vi "pulse Tx 2 spc.vi"(9 "enable line":bool=TRUE, 10 "take it!":bool, 11 "Cluster":T2={"PW"=0, "frequency shift"=0.0, "amp"=0.9999923706054688, "mode type"=enum."CW", "mode depth"=0, "mode filter"=0, "phase shift"=0.0, "pulse shape filter"=0}) -> (0 "output valid":bool, 1 "IQ out":T1[](array[typedef]), 2 "free dds":bool, 4 "frequncy":fxp<+/-,48,0>, 6 "phase":fxp<+/-,16,1>)   [LabVIEW 2021]
uses:
  pulse_tx_vis/pdw.ctl
  pulse_tx_vis/CTL/mode_type.ctl
  <instrlib>/_niInstr/DSP/v1/Shared/Public/IQ Data.ctl
  <instrlib>/_niInstr/DSP/v1/FPGA/Public/Sub VIs/Frequency Shift/Frequency Shift - 2 spc.vi
  <instrlib>/_niInstr/Basic Elements/v1/FPGA/Private/Count Up U32.vi
  <vilib>/rvi/FXPMathLib/FxpAdd/XNode/nifxpmath_Add.xnode
  <instrlib>/_niInstr/DSP/v1/Shared/niInstr DSP v1 Shared.lvlib
  <instrlib>/_niInstr/Basic Elements/v1/FPGA/niInstr Basic Elements v1 FPGA.lvlib
  <vilib>/rvi/FXPMathLib/sim/FxpSim.dll
  <instrlib>/_niInstr/DSP/v1/FPGA/niInstr DSP v1 FPGA.lvlib
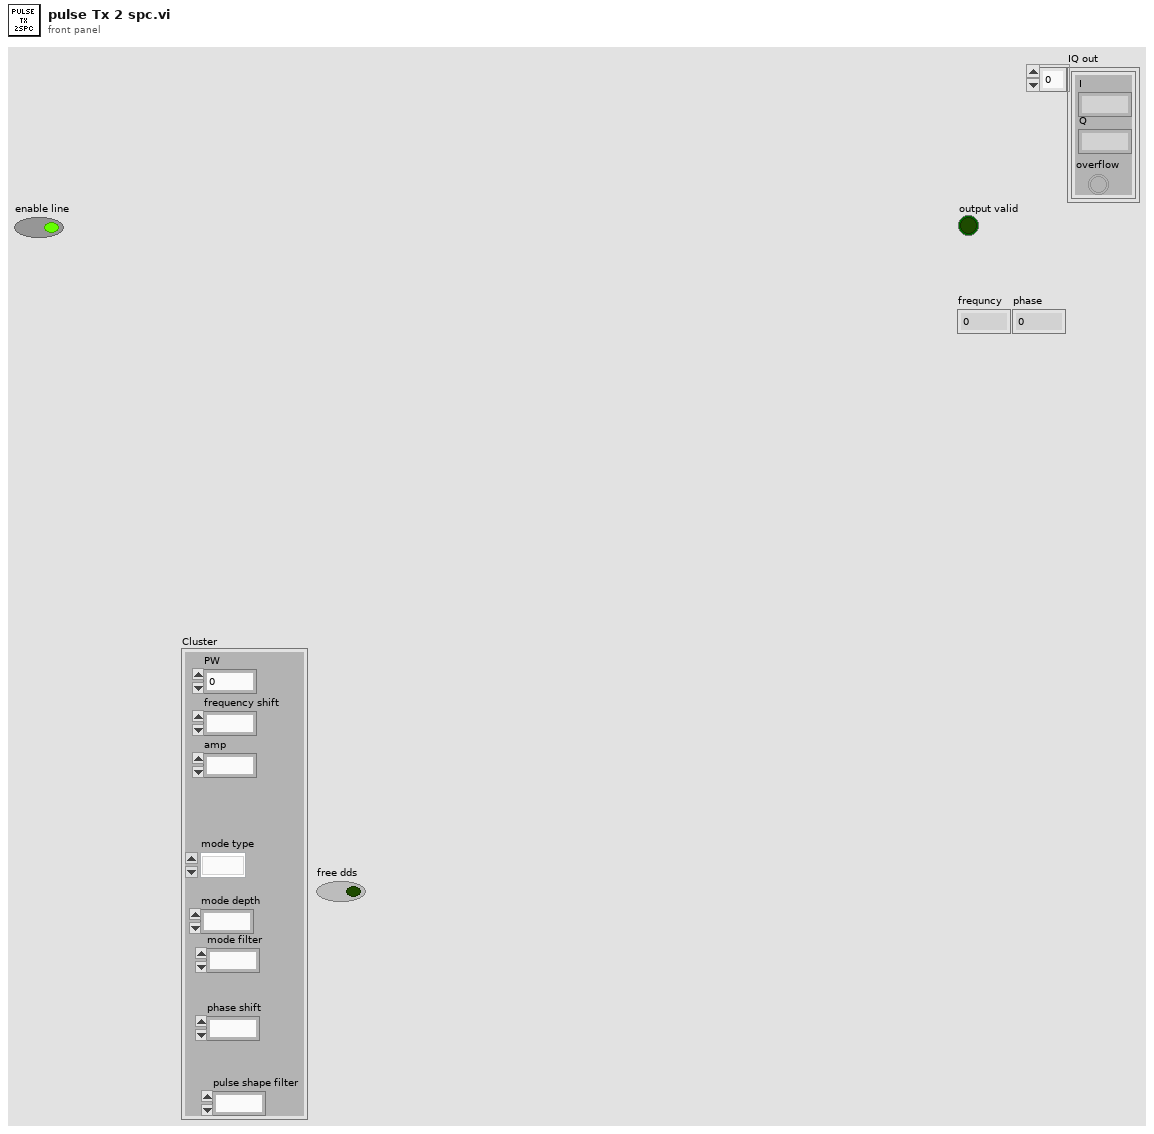
[diagram p1: front panel]
types:
  T1 = typedef "niInstr DSP v1 Shared.lvlib/IQ Data.ctl" = cluster{"I":fxp<+/-,18,1>, "Q":fxp<+/-,18,1>, "overflow":bool}
  T2 = typedef "pdw.ctl" = cluster{"PW":u32, "frequency shift":fxp<+/-,48,0>, "amp":fxp<+/-,18,1>, "mode type":T3, "mode depth":u32, "mode filter":u8, "phase shift":fxp<+/-,16,1>, "pulse shape filter":u8}
  T3 = typedef "mode_type.ctl" = enum8{"CW", "from memory 1", "NC - cw", "LFM", "BPSK", "QPSK"}
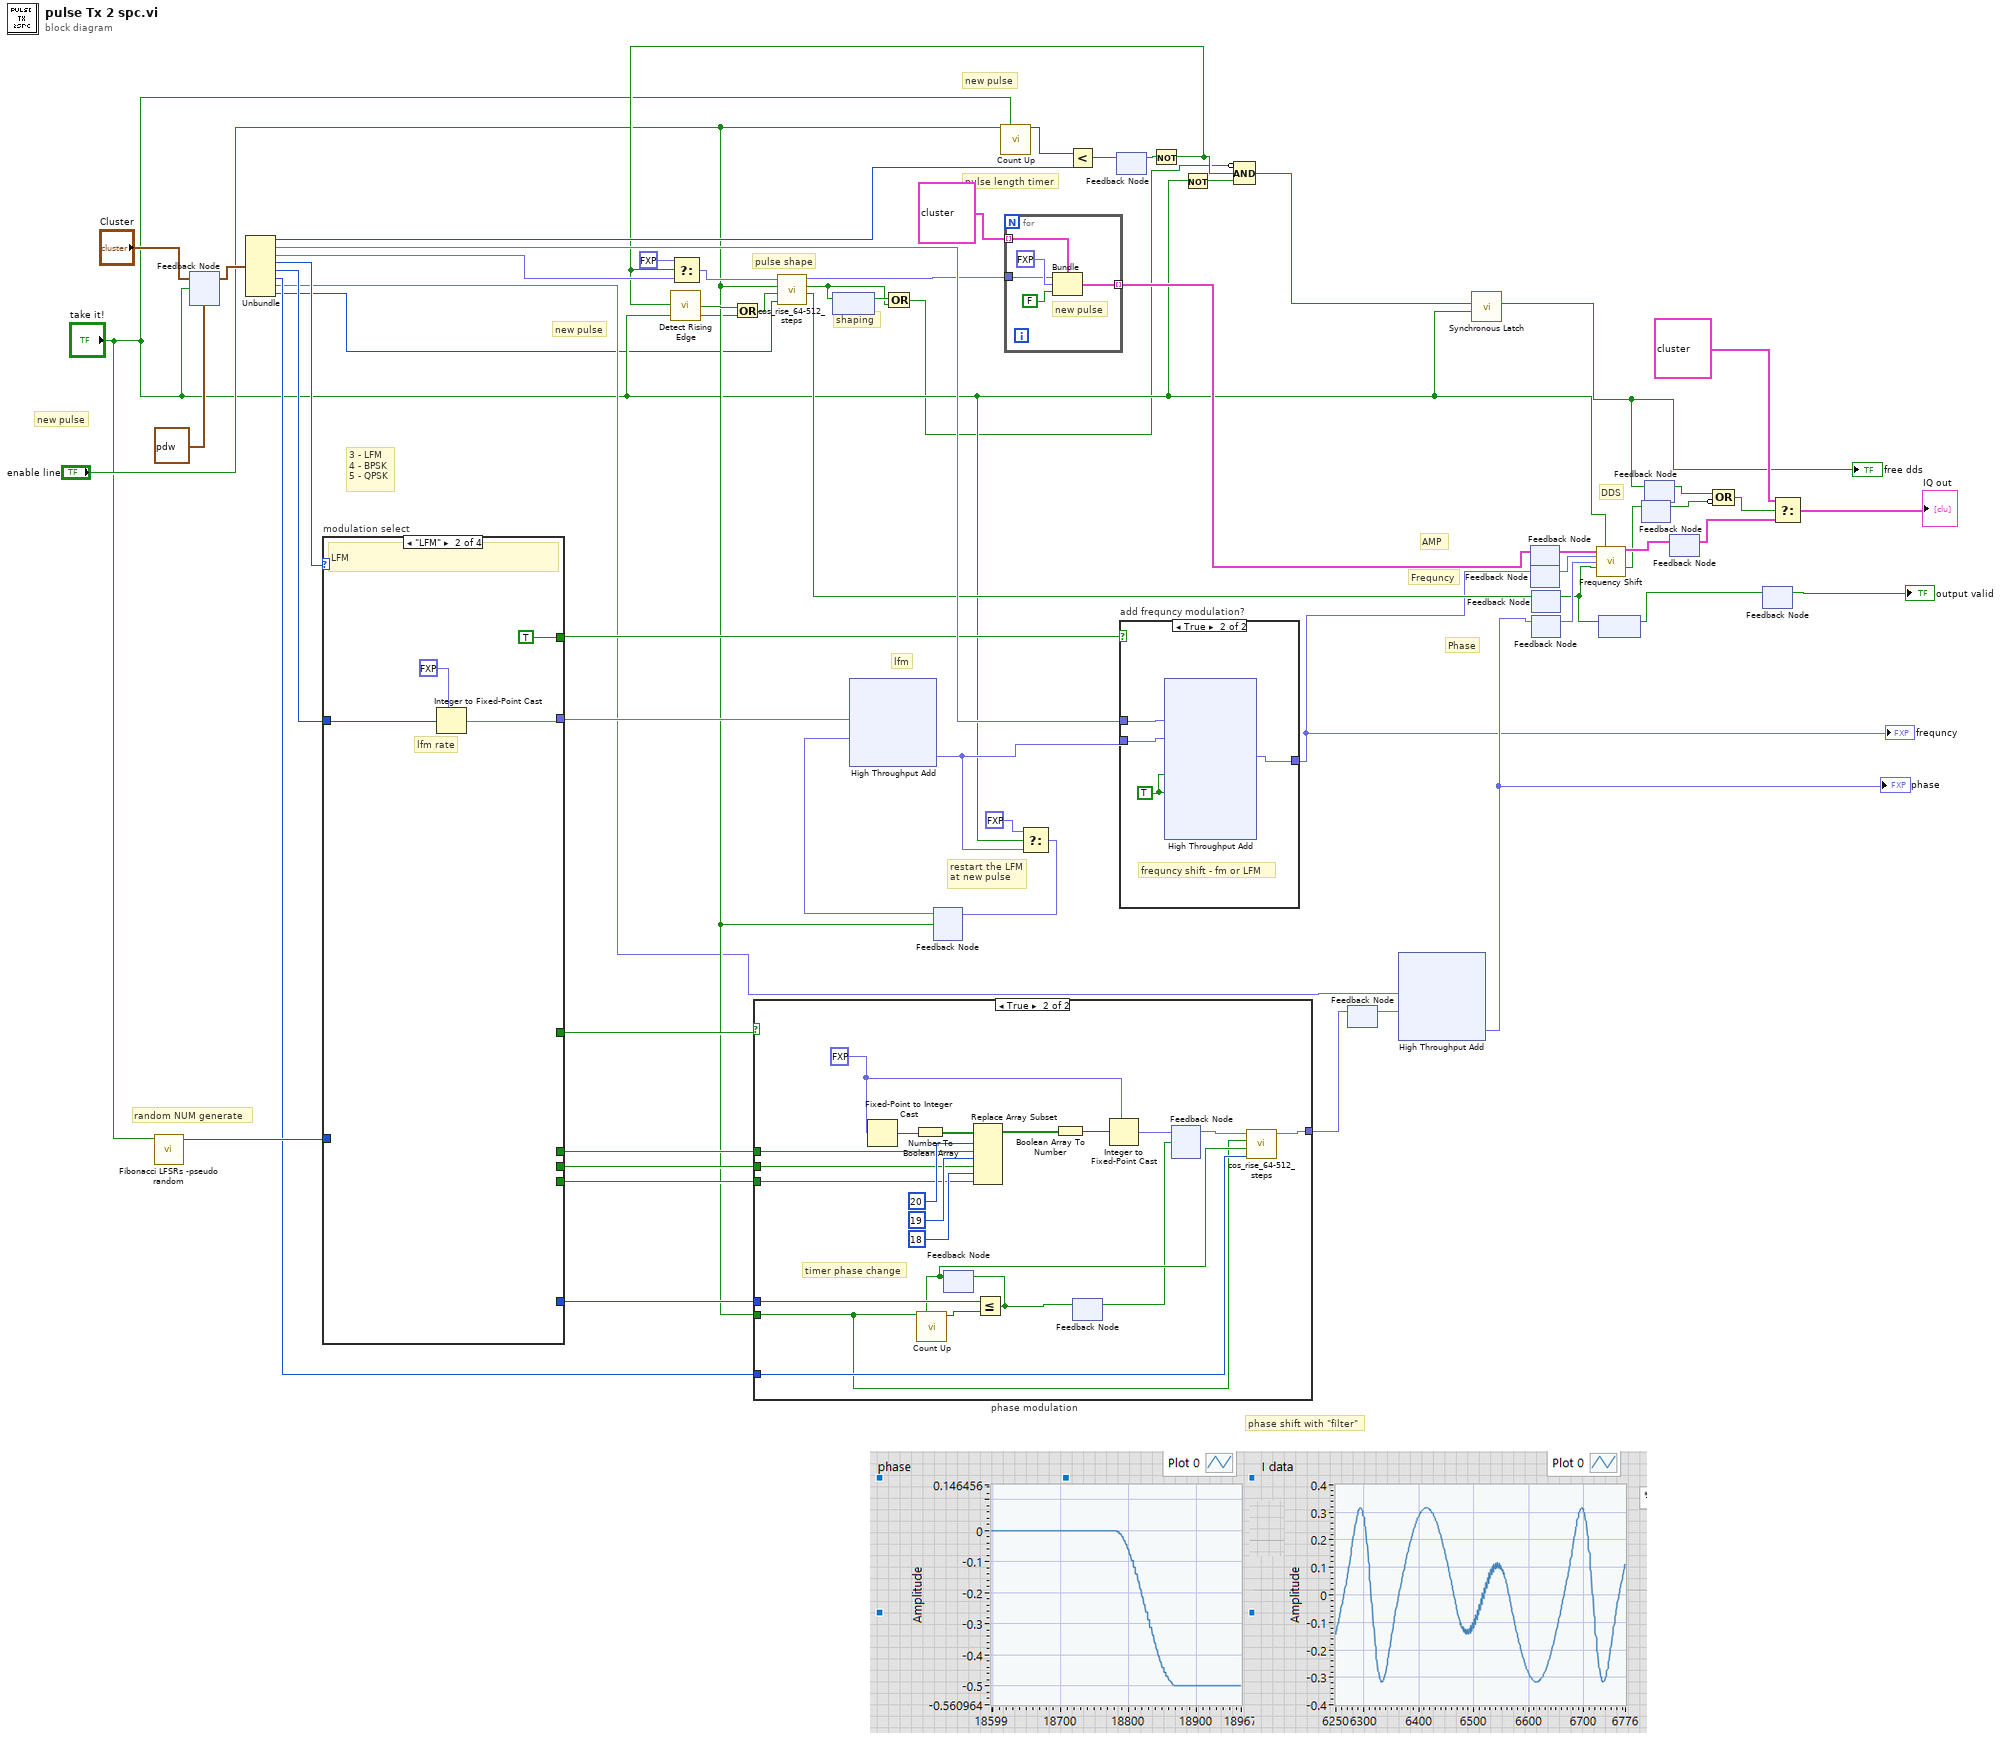
[diagram p0: block diagram]
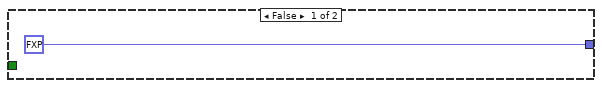
[diagram p2: hidden frame]
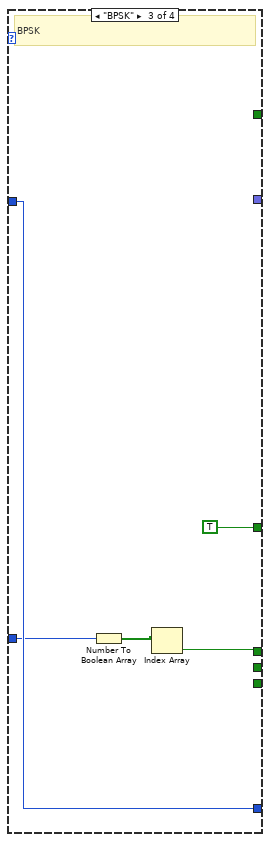
[diagram p5: hidden frame]
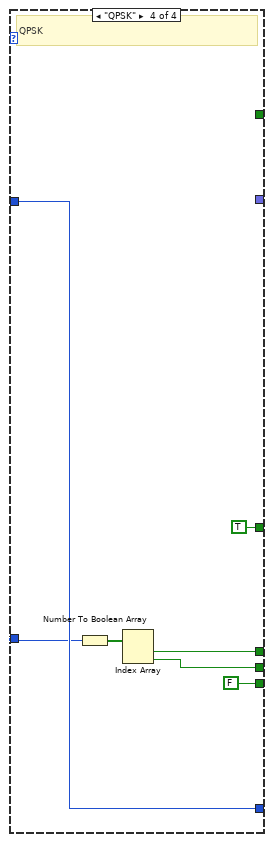
[diagram p6: hidden frame]
diagram:
  # "random NUM generate"
  # "phase shift with \"filter\""
  # "Phase"
  # "Frequncy"
  # "AMP"
  # "DDS"
  # "shaping"
  # "3 - LFM\n4 - BPSK\n5 - QPSK"
  # "pulse length timer"
  # "restart the LFM\nat new pulse"
  # "lfm"
  # "pulse shape"
  # "new pulse"
  # "new pulse"
  # "new pulse"
  n1 = call "Fibonacci LFSRs -pseudo random.vi"("reset random"="take it!") -> ("rand number"=w36:u16)  [unwired: 10 in]
  n2 = feedback #1(T2 {"PW"=0, "frequency shift"=0.0, "amp"=0.9999923706054688, "mode type"=enum."CW", "mode depth"=0, "mode filter"=0, "phase shift"=0.0, "pulse shape filter"=0} ("Cluster")) -> (w59:T2)
  n3 = feedback-in #1("Cluster", "take it!") -> ()
  n4 = Unbundle(w59) -> ("PW"=w61:u32, "frequency shift"=w55:fxp<+/-,48,0>, "amp"=w39:fxp<+/-,18,1>, "mode type"=w56:T3, "mode depth"=w31:u32, "mode filter"=w30:u8, "phase shift"=w28:fxp<+/-,16,1>, "pulse shape filter"=w13:u8)
  n5 = case "modulation select" shown="\"LFM\"" w56 {
    tunnel: w31 -> [_ w64 w67 w72]
    tunnel: [_ w63 _ _] -> w52
    tunnel: [_ TRUE ("s") _ _] -> w49
    tunnel: [_ _ _ FALSE] -> w47
    tunnel: [_ _ _ w74] -> w46
    tunnel: [_ _ w69 w76] -> w45
    tunnel: [_ _ TRUE TRUE] -> w44
    tunnel: [_ _ w67 w72] -> w43
    tunnel: w36 -> [_ _ w66 w71]
    frame Default {
    }
    frame "LFM" {
      # "lfm rate"
      # "LFM"
      n6 = Integer to Fixed-Point Cast(fixed-point type=fxp<+/-,32,-16> 0.0, integer=w64) -> (fixed-point=w63:fxp<+/-,32,-16>)
    }
    frame "BPSK" {
      # "BPSK"
      n7 = Number To Boolean Array(number=w66) -> (Boolean array=w70:bool[])
      n8 = Index Array(array=w70) -> (element=w69:bool)  [unwired: 1 in]
    }
    frame "QPSK" {
      # "QPSK"
      n9 = Number To Boolean Array(number=w71) -> (Boolean array=w77:bool[])
      n10 = Index Array(array=w77) -> (element #1=w76:bool, element #2=w74:bool)  [unwired: 2 in]
    }
  }
  n11 = case "phase modulation" shown="True" w44 {
    tunnel: w47 -> [_ w91]
    tunnel: w46 -> [_ w90]
    tunnel: w45 -> [_ w89]
    tunnel: w43 -> [_ w87]
    tunnel: [fxp<+/-,16,1> 0.0 ("filter out") w84] -> w15
    tunnel: w30 -> [_ w82]
    tunnel: "enable line" -> [_ w81]
    frame False {
    }
    frame True {
      w93 = fxp<+/-,21,0> 0.0 ("phase")
      # "timer phase change"
      n12 = Fixed-Point to Integer Cast(1:w93) -> (0:w99:i32)
      n13 = Number To Boolean Array(number=w99) -> (Boolean array=w97:bool[])
      n14 = feedback #2() -> (w83:bool)  [unwired: 1 in]
      n15 = call-poly <instrlib>:"Count Up.vi"("increment"=w81, "reset"=w83) -> ("count out"=w86:u32)  [unwired: 13 in]
      n16 = Replace Array Subset(array=w97, new element #1=w89, index #1=20 ("index"), new element #2=w90, index #2=19 ("index"), new element #3=w91, index #3=18 ("index")) -> (w92:bool[])
      n17 = Less Or Equal?(x=w87, y=w86) -> (x <= y?=w80:bool)
      n18 = feedback-in #2(w80) -> ()
      n19 = Boolean Array To Number(Boolean array=w92) -> (number=w98:u32)
      n20 = feedback-in #3(w80) -> ()
      n21 = feedback #3() -> (w79:bool)  [unwired: 1 in]
      n22 = Integer to Fixed-Point Cast(fixed-point type=w93, integer=w98) -> (fixed-point=w88:fxp<+/-,21,0>)
      n23 = feedback-in #4(w88, w79) -> ()
      n24 = feedback #4() -> (w85:fxp<+/-,21,0>)  [unwired: 1 in]
      n25 = call "cos_rise_64-512_steps.vi"("filter select"=w82, "new step"=w83, "run"=w81, "data in"=w85) -> ("data out"=w84:fxp<+/-,16,1>)  [unwired: 5 in, 2 out]
    }
  }
  n26 = feedback #5() -> (w3:bool)  [unwired: 1 in]
  n27 = feedback #6() -> (w51:fxp<+/-,48,0>)  [unwired: 1 in]
  n28 = xnode ("High Throughput Add")("x"=w52, "y"=w51) -> ("x+y"=w50:fxp<+/-,48,0>)
  n29 = call-poly <instrlib>:"Count Up.vi"("increment"="enable line", "reset"="take it!") -> ("count out"=w42:u32)  [unwired: 13 in]
  n30 = Select(t=fxp<+/-,48,0> 0.0, s="take it!", f=w50) -> (s? t:f=w53:fxp<+/-,48,0>)
  n31 = feedback-in #6(w53, "enable line") -> ()
  n32 = Less?(x=w42, y=w61) -> (x < y?=w41:bool)
  n33 = feedback #7() -> (w40:bool)  [unwired: 1 in]
  n34 = feedback-in #7(w41) -> ()
  n35 = case "add frequncy modulation?" shown="True" w49 {
    tunnel: w55 -> [w100 w104]
    tunnel: w50 -> [_ w103]
    tunnel: [w100 w102] -> w25
    frame False {
    }
    frame True {
      w101 = TRUE ("input valid")
      # "frequncy shift - fm or LFM"
      n36 = xnode ("High Throughput Add")("x"=w104, "y"=w103, "input valid"=w101, "ready for output (T)"=w101) -> ("x+y"=w102:fxp<+/-,48,0>)  [unwired: 2 out]
    }
  }
  "frequncy" <- w25
  n37 = Not(x=w40) -> (.not. x?=w33:bool)
  n38 = call <instrlib>:"Detect Rising Edge.vi"("signal"=w33) -> ("edge detected"=w32:bool)  [unwired: 14 in]
  n39 = Select(t=fxp<+/-,18,1> 0.0, s=w33, f=w39) -> (s? t:f=w38:fxp<+/-,18,1>)
  n40 = Or(x=w32, y="take it!") -> (x .or. y?=w34:bool)
  n41 = call "cos_rise_64-512_steps.vi"("filter select"=w13, "new step"=w34, "run"="enable line", "data in"=w38) -> ("output valid"=w26:bool, "steping"=w2:bool, "data out"=w35:fxp<+/-,16,1>)  [unwired: 5 in]
  n42 = feedback-in #5(w2) -> ()
  n43 = Or(x=w3, y=w2) -> (x .or. y?=w1:bool)
  n44 = for {
    tunnel: w35 -> [w107]
    tunnel: [w106] -> w24 mode=indexing
    tunnel: T1[] [{"I"=0.0, "Q"=0.0, "overflow"=FALSE}, {"I"=0.0, "Q"=0.0, "overflow"=FALSE}] ("t") -> [w105] mode=indexing
    # "new pulse"
    n45 = Bundle(cluster=w105, "I"=w107, "Q"=fxp<+/-,18,1> 0.0, "overflow"=FALSE ("input valid")) -> (w106:T1)
  }
  n46 = Not(x="take it!") -> (.not. x?=w58:bool)
  n47 = Compound Arithmetic op=AND(invert w1, w33, w58) -> (w57:bool)
  n48 = feedback-in #8(w15) -> ()
  n49 = feedback #8() -> (w14:fxp<+/-,16,1>)  [unwired: 1 in]
  n50 = xnode ("High Throughput Add")("x"=w28, "y"=w14) -> ("x+y"=w27:fxp<+/-,16,1>)
  "phase" <- w27
  n51 = call <instrlib>:"Synchronous Latch.vi"("clear"="take it!", "set"=w57) -> ("out"=w5:bool)  [unwired: 9 in]
  "free dds" <- w5
  n52 = feedback #9() -> (w18:T1[])  [unwired: 1 in]
  n53 = feedback-in #9(w24) -> ()
  n54 = feedback #10() -> (w22:fxp<+/-,48,0>)  [unwired: 1 in]
  n55 = feedback-in #10(w25) -> ()
  n56 = feedback #11() -> (w10:bool)  [unwired: 1 in]
  n57 = feedback-in #11(w26) -> ()
  n58 = feedback-in #12(w27) -> ()
  n59 = feedback #12() -> (w21:fxp<+/-,16,1>)  [unwired: 1 in]
  n60 = call-poly <instrlib>:"Frequency Shift.vi"("data in"=w18, "reset"="take it!", "frequency shift"=w22, "phase"=w21, "input valid"=w10) -> ("data out"=w17:T1[], "output valid"=w7:bool)  [unwired: 7 in, 2 out]
  n61 = feedback #13() -> (w9:bool)  [unwired: 1 in]
  n62 = feedback-in #13(w10) -> ()
  n63 = feedback #14() -> (w6:bool)  [unwired: 1 in]
  n64 = feedback-in #14(w7) -> ()
  n65 = feedback #15() -> (w4:bool)  [unwired: 1 in]
  n66 = feedback-in #15(w5) -> ()
  n67 = feedback #16() -> (w16:T1[])  [unwired: 1 in]
  n68 = feedback-in #16(w17) -> ()
  n69 = Compound Arithmetic op=OR(w4, invert w6) -> (w12:bool)
  n70 = feedback #17() -> (→"output valid":bool)  [unwired: 1 in]
  n71 = feedback-in #17(w9) -> ()
  n72 = Select(t=T1[] [{"I"=0.0, "Q"=0.0, "overflow"=FALSE}, {"I"=0.0, "Q"=0.0, "overflow"=FALSE}], s=w12, f=w16) -> (s? t:f=→"IQ out":T1[])
